vi "Generate Command Frame Vectors.vi"(0 "RFFE Extended Command in":refnum<class "RFFE Extended Command.lvclass">, 11 "error in (no error)":errorcluster) -> (4 "RFFE Extended Command out":refnum<class "RFFE Extended Command.lvclass">, 6 "Command Frame Vectors":string[](array[string]), 15 "error out":errorcluster)   [LabVIEW 2018, in "MIPI RFFE API.lvlib" / "RFFE Extended Command.lvclass"]
uses:
  RFFE Extended Command.lvclass
  C:/Users/semoore/Projects/mipi-rffe-labview-oop/Command/RFFE Command.lvclass
  Command/Get Slave Address Field Width.vi
  Get Byte Count Field Width.vi
  Command/RFFE Command.lvclass
  MIPI RFFE API.lvlib
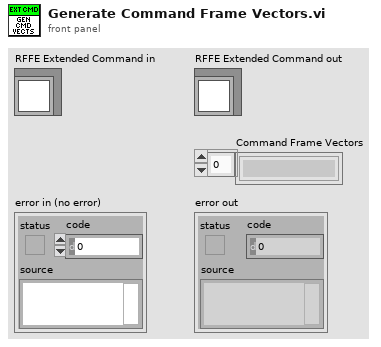
[diagram p1: front panel]
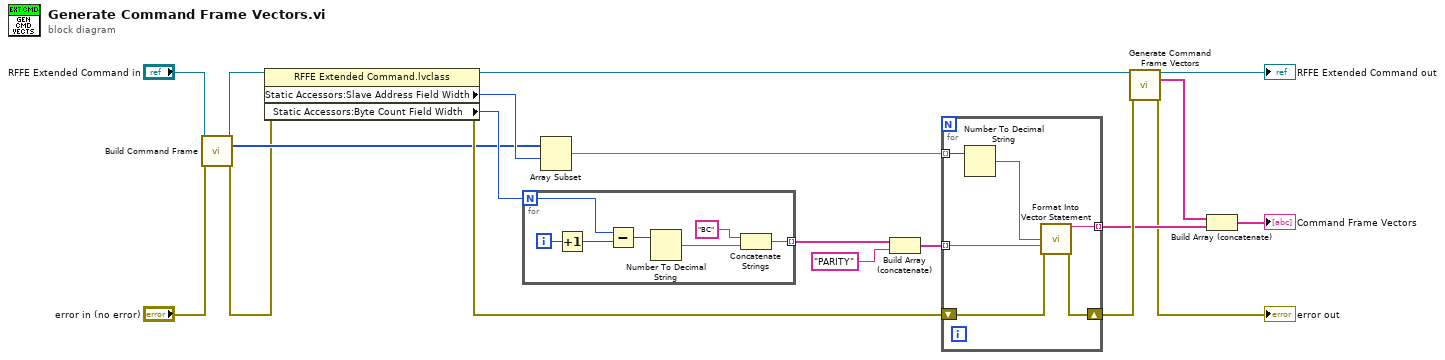
[diagram p0: block diagram]
diagram:
  n1 = call-dynamic "Build Command Frame.vi"("RFFE Extended Command in"="RFFE Extended Command in", "error in (no error)"="error in (no error)") -> ("RFFE Extended Command out"=w4:refnum<class "RFFE Extended Command.lvclass">, "Command Frame"=w3:u8[], "error out"=w1:errorcluster)  [unwired: 11 in]
  n2 = property class="RFFE Extended Command.lvclass"(reference=w4, error in=w1) -> (reference out=w9:refnum<class "RFFE Extended Command.lvclass">, error out=w11:errorcluster, "Static Accessors:Slave Address Field Width"=w19:i32, "Static Accessors:Byte Count Field Width"=w18:i32)
  n3 = for {
    N: w18 -> [w24]
    tunnel: [w20] -> w16 mode=indexing
    i -> [w26]
    n4 = Increment(x=w26) -> (x+1=w25:i32)
    n5 = Subtract(x=w24, y=w25) -> (x-y=w23:i32)
    n6 = Number To Decimal String(number=w23) -> (decimal integer string=w22:string)  [unwired: 1 in]
    n7 = Concatenate Strings("BC", w22) -> (w20:string)
  }
  n8 = Array Subset(array=w3, index=w19) -> (w13:u8[])  [unwired: 1 in]
  n9 = Build Array (concatenate)(w16, "PARITY" ("format string")) -> (w14:string[])
  n10 = for {
    tunnel: w14 -> [w32] mode=indexing
    tunnel: w13 -> [w31] mode=indexing
    shift-right: [w30] -> w12
    shift-left: w11 -> [w29]
    tunnel: [w28] -> w10 mode=indexing
    n11 = Number To Decimal String(number=w31) -> (decimal integer string=w27:string)  [unwired: 1 in]
    n12 = call "Format Into Vector Statement.vi"("DATA (0)"=w27, "Comment"=w32, "error in (no error)"=w29) -> ("Vector Statement"=w28:string, "error out"=w30:errorcluster)  [unwired: 11 in]
  }
  n13 = call-parent "Generate Command Frame Vectors.vi"("RFFE Command in"=w9, "error in (no error)"=w12) -> ("RFFE Command out"=→"RFFE Extended Command out":refnum<class "RFFE Extended Command.lvclass">, "Command Frame Vectors"=w17:string[], "error out"=→"error out":errorcluster)  [unwired: 11 in]
  n14 = Build Array (concatenate)(w17, w10) -> (→"Command Frame Vectors":string[])
